vi "configure_scaffold.vi"(8 "error in (no error)":errorcluster, 10 "visibilities":T1, 11 "ScanModeDL090923Scaffold in":refnum<class "ImagingModeDL090923Scaffold.lvclass">) -> (0 "error out":errorcluster, 3 "ScanModeDL090923Scaffold out":refnum<class "ImagingModeDL090923Scaffold.lvclass">)   [LabVIEW 2010, in "ImagingModeDL090923Scaffold.lvclass"]
uses:
  ImagingModeDL090923Scaffold.lvclass
  configuration_visibility_cluster.ctl
  component_configuration_visibility_cluster.ctl
  common/xcontrols/XComponentSpecification/XComponentSpecification/XComponentSpecification.xctl
  ImagingModeDL090923Scaffold.lvclass/ImagingModeDL090923Scaffold.ctl
  Stimulator/GenericStimulator/GenericStimulator/GenericStimulator.lvclass
  Analyser/GenericAnalyser/GenericAnalyser/GenericAnalyser.lvclass
  Display/GenericDisplay/GenericDisplay/GenericDisplay.lvclass
  DataCollection/GenericDataCollection/GenericDataCollection/GenericDataCollection.lvclass
  ImageAssembler/GenericImageAssembler/GenericImageAssembler/GenericImageAssembler.lvclass
  DAQ/GenericDAQ/GenericDAQ/GenericDAQ.lvclass
  ScanHead/GenericScanHead/GenericScanHead/GenericScanHead.lvclass
  Trajectory/GenericTrajectory/GenericTrajectory/GenericTrajectory.lvclass
  Instrument/GenericInstrument/GenericInstrument/GenericInstrument.lvclass
  common/classes/ErrorController/ErrorController/class_data.vi
  common/classes/GenericComponent/GenericComponent/GenericComponent.lvclass
  common/classes/ErrorController/ErrorController/ErrorController.lvclass
panel:
  out "LSID":string
  in  "Tab Control":T3(tab)
  in  "Instrument adapter path":path caption="adapter path"
  in  "instrument spec":T4(xcontrol)
  in  "Trajectory adapter path":path caption="adapter path"
  in  "trajectory spec":T4(xcontrol)
  in  "ScanHead adapter path":path caption="adapter path"
  in  "scanHead spec":T4(xcontrol)
  in  "DAQ adapter path":path caption="adapter path"
  in  "daq spec":T4(xcontrol)
  in  "ImageAssembler adapter path":path caption="adapter path"
  in  "Trajectory-to-ImageAssembler adapter":path caption="trajectory-to-image-assembler adapter (has to be compatible with both the trajectory and the image assembler you have chosen!)"
  in  "imageAssembler spec":T4(xcontrol)
  in  "DataCollection adapter path":path caption="adapter path"
  in  "dataCollection spec":T4(xcontrol)
  in  "Display adapter path":path caption="adapter path"
  in  "display spec":T4(xcontrol)
  in  "Analyser adapter path":path caption="adapter path"
  in  "analyser spec":T4(xcontrol)
  in  "Stimulator adapter path":path caption="adapter path"
  in  "stimulator spec":T4(xcontrol)
  in  "save":bool
  in  "cancel":bool
  out "Configuration":string
  # "Configure ImagingMode"
  # "The ImagingMode component is the central component that determines how images are acquired. It determines also all other top-level components which have to be defined on this configuration dialog (see other tabs)."
  # "The Instrument component can control and/or hold information about accessory devices and hardware component."
  # "In laser-scanning-based imagingModes, the Trajectory component defines how the laser focal point is moved through the sample."
  # "In laser-scanning-based imagingModes, the ScanHead component controls the invididual laser scanners."
  # "The DAQ component is responsible for reading in image data (either as a stream of pixels in laser-scanning-based ImagingModes, or as images in the case of camera-based ImagingModes)."
  # "The ImageAssembler if responsible for assembling pixels streams into whole images and/or refinement of these images."
  # "The DataCollection component is responsible for storing images permanently to disk."
  # "The Display component is responsible for displaying images to the users."
  # "The Analyser component is responsible for analysing image streams. \n\nNote: Leave the input fields below empty if you are not interested in on-line analysis of acquired images."
  # "The Stimulator component can deliver stimuli to the sample being imaged. \n\nNote: leave the input fields below empty if you don't want to control a stimulator device with HelioScan."
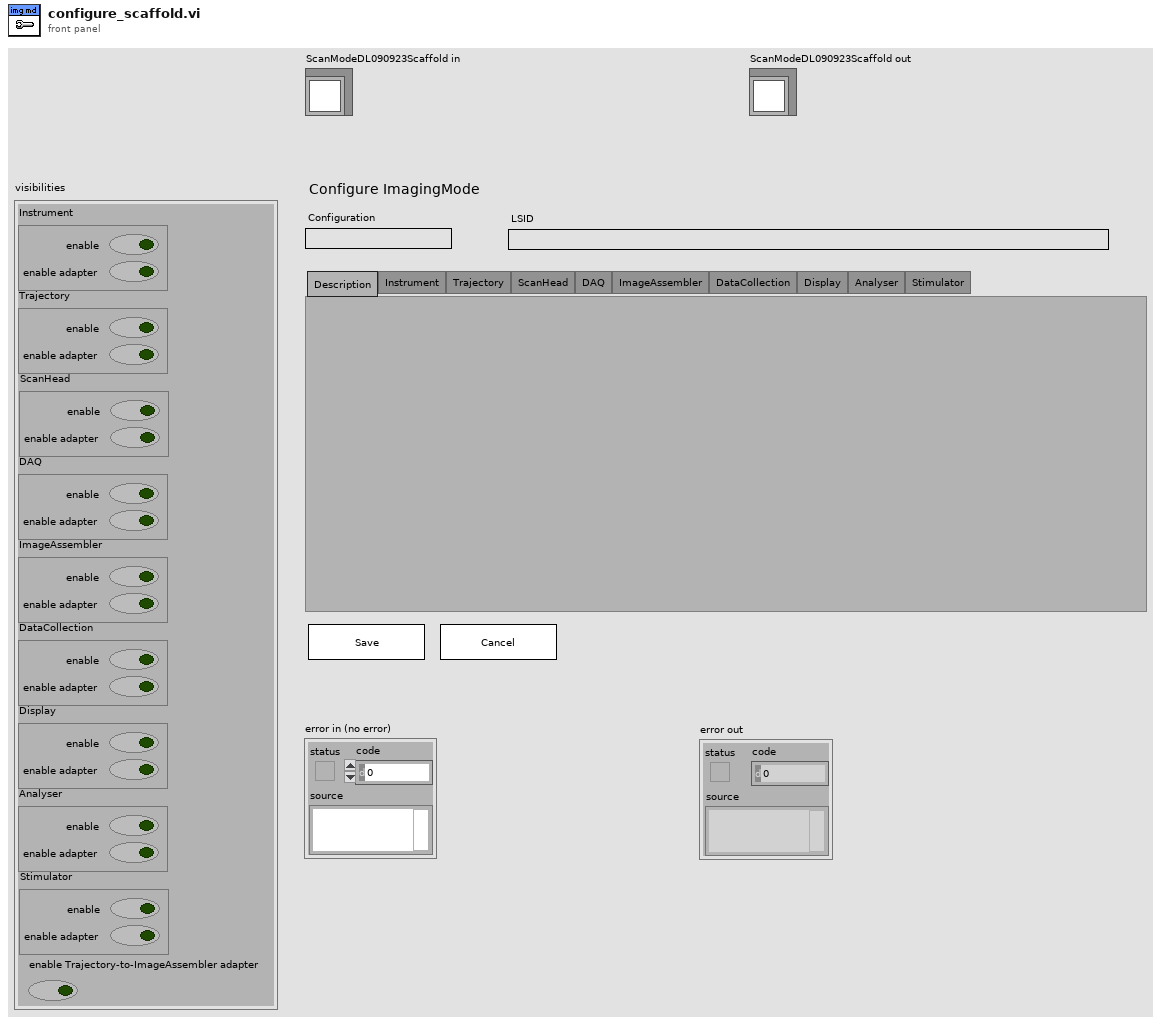
[diagram p1: front panel]
types:
  T1 = typedef "ImagingModeDL090923Scaffold.lvclass/configuration_visibility_cluster.ctl" = cluster{"Instrument":T2, "Trajectory":T2, "ScanHead":T2, "DAQ":T2, "ImageAssembler":T2, "DataCollection":T2, "Display":T2, "Analyser":T2, "Stimulator":T2, "enable Trajectory-to-ImageAssembler adapter":bool}
  T2 = typedef "ImagingModeDL090923Scaffold.lvclass/component_configuration_visibility_cluster.ctl" = cluster{"enable":bool, "enable adapter":bool}
  T3 = enum32{"Description", "Instrument", "Trajectory", "ScanHead", "DAQ", "ImageAssembler", "DataCollection", "Display", "Analyser", "Stimulator"}
  T4 = cluster{"class path":string, "configuration":string, "label":string, "settings name":string}
  T5 = typedef "LSID_cluster.ctl" = cluster{"identifier":string, "revision":i32}
  T6 = typedef "plugin_specification.ctl" = cluster{"class path":string, "configuration":string, "label":string, "settings name":string}
  T7 = typedef "ImagingModeDL090923Scaffold.lvclass/config_data_cluster.ctl" = cluster{"Instrument":T8, "Trajectory":T8, "ScanHead":T8, "DAQ":T8, "ImageAssembler":T8, "DataCollection":T8, "Display":T8, "Analyser":T8, "Stimulator":T8, "Trajectory-to-ImageAssembler adapter path":string, "LSID (cluster)":T5, "special":string}
  T8 = typedef "ImagingModeDL090923Scaffold.lvclass/component_specification_cluster.ctl" = cluster{"specification":T6, "adapter path":string}
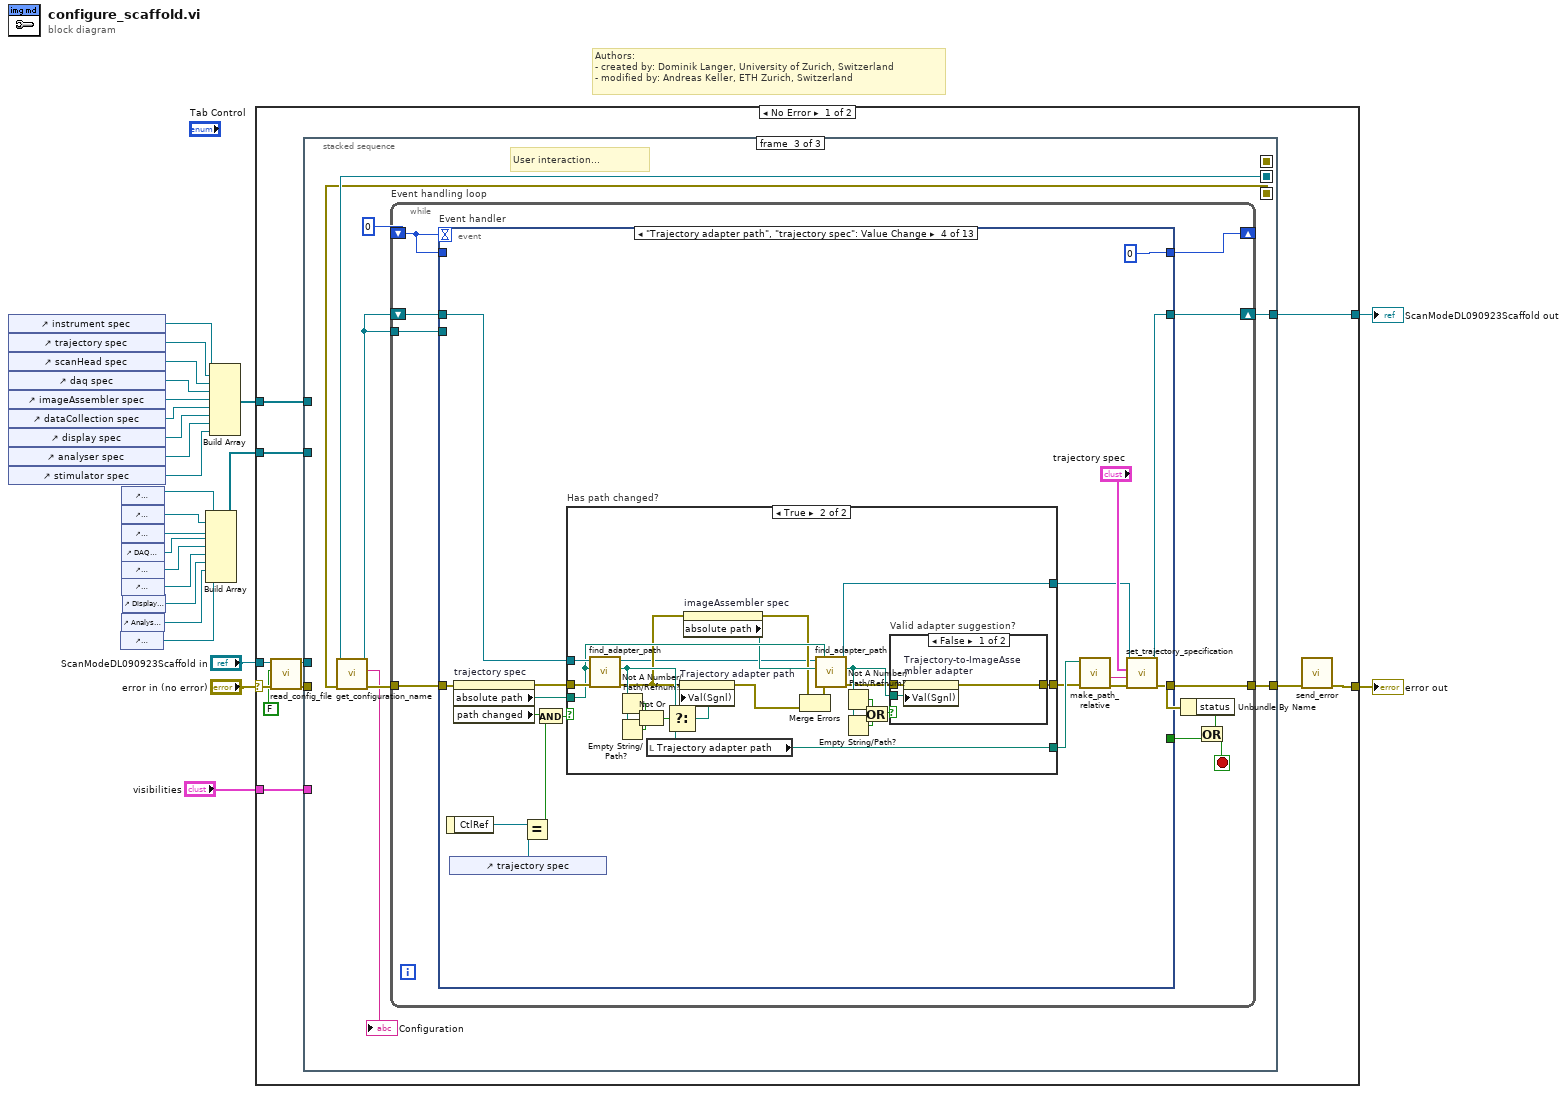
[diagram p0: block diagram]
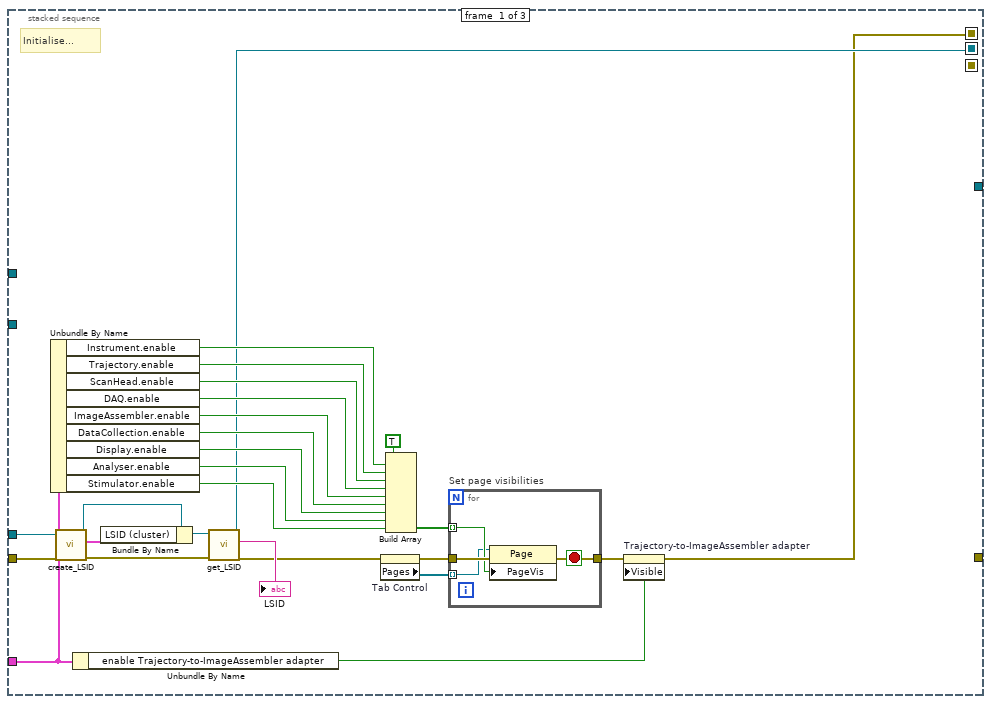
[diagram p2: hidden frame]
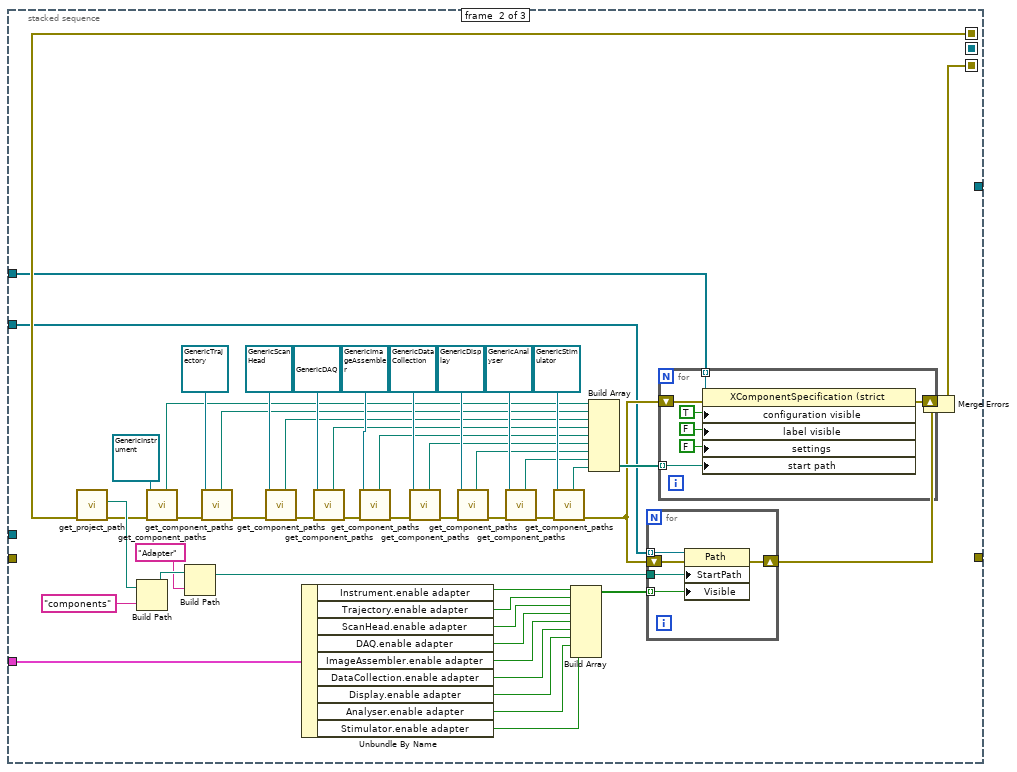
[diagram p3: hidden frame]
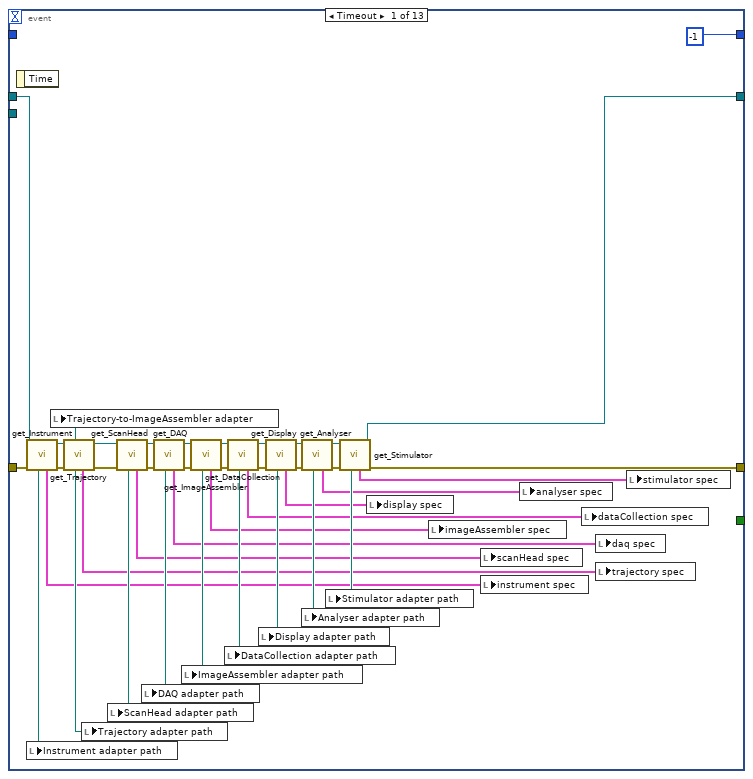
[diagram p4: hidden frame]
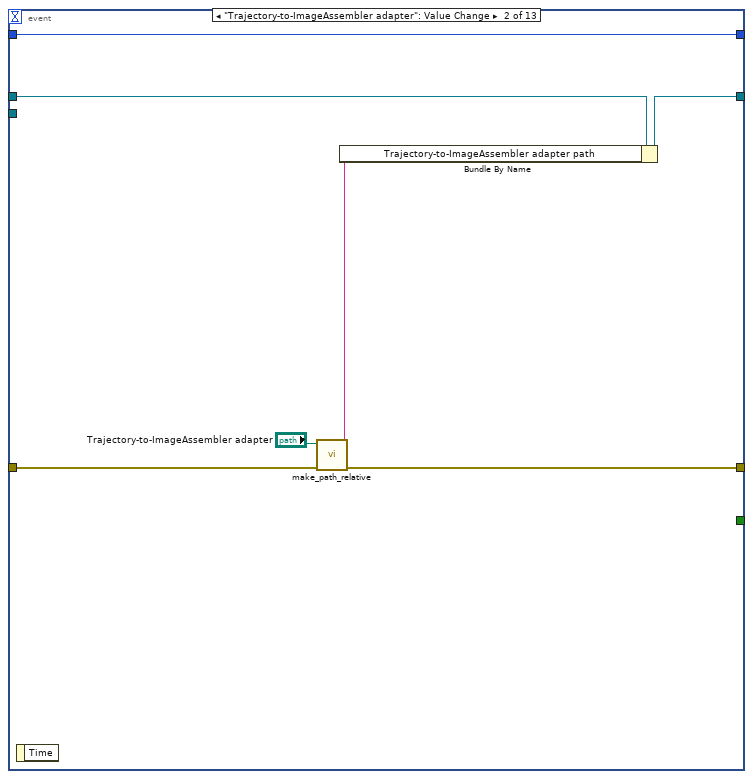
[diagram p5: hidden frame]
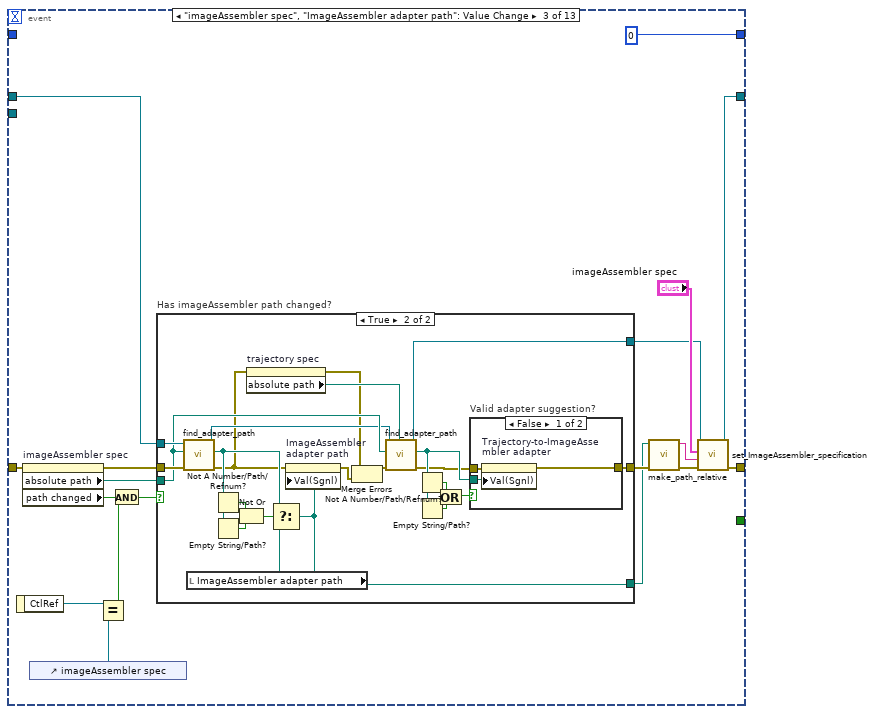
[diagram p6: hidden frame]
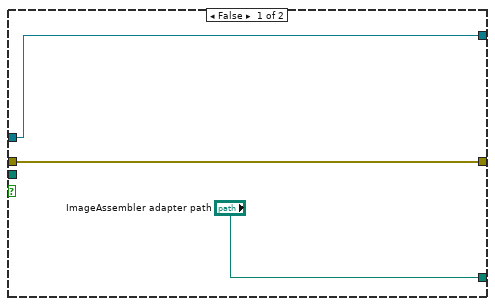
[diagram p7: hidden frame]
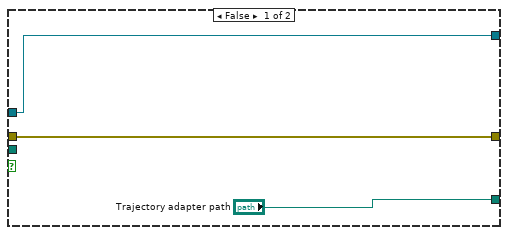
[diagram p9: hidden frame]
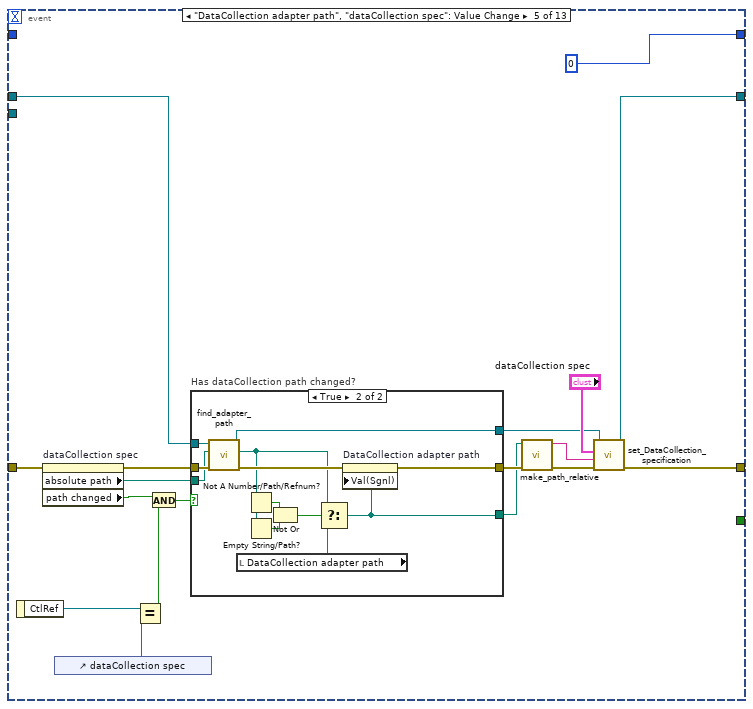
[diagram p11: hidden frame]
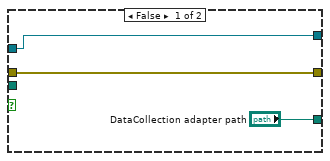
[diagram p12: hidden frame]
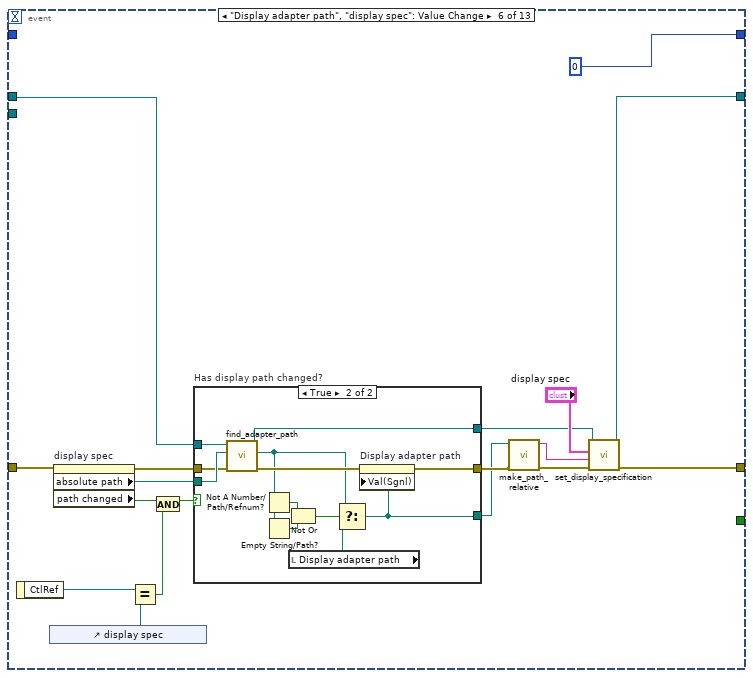
[diagram p13: hidden frame]
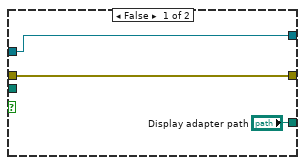
[diagram p14: hidden frame]
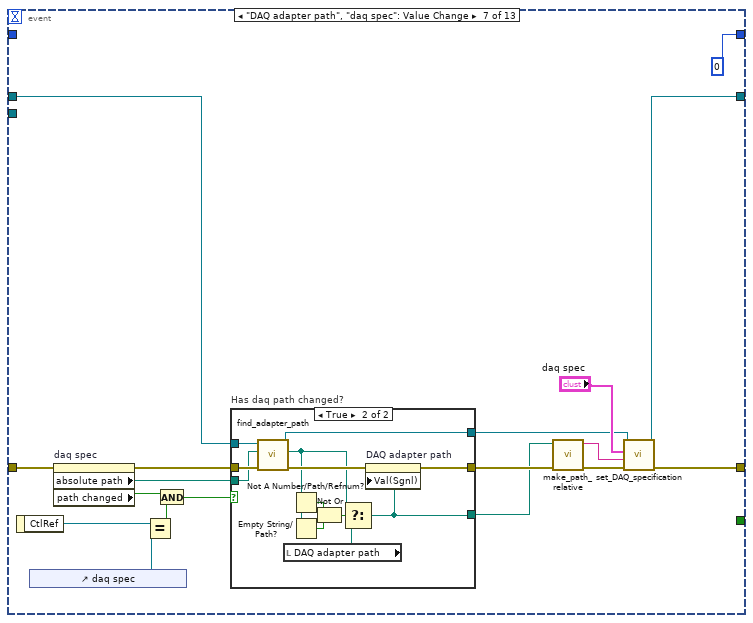
[diagram p15: hidden frame]
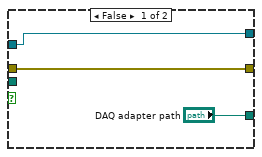
[diagram p16: hidden frame]
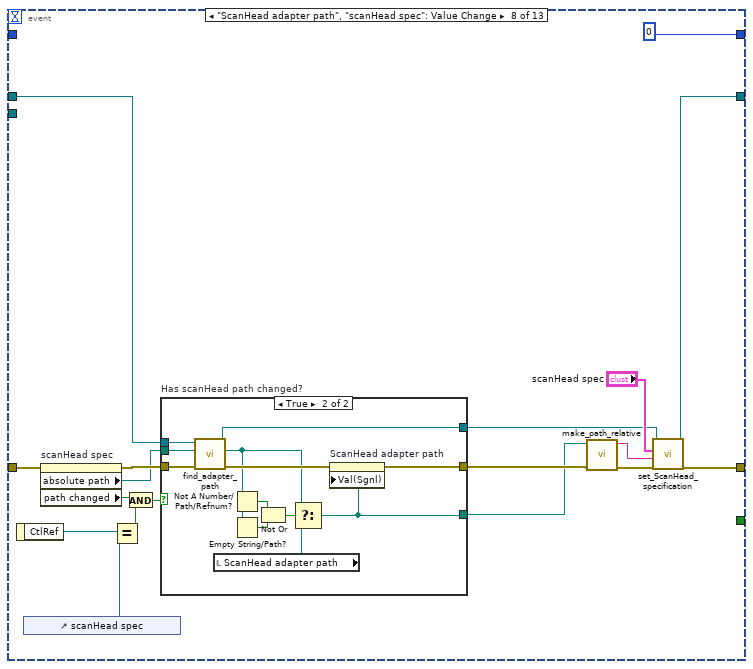
[diagram p17: hidden frame]
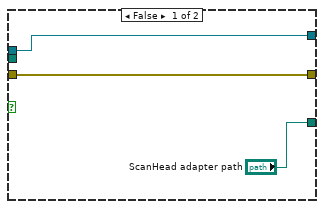
[diagram p18: hidden frame]
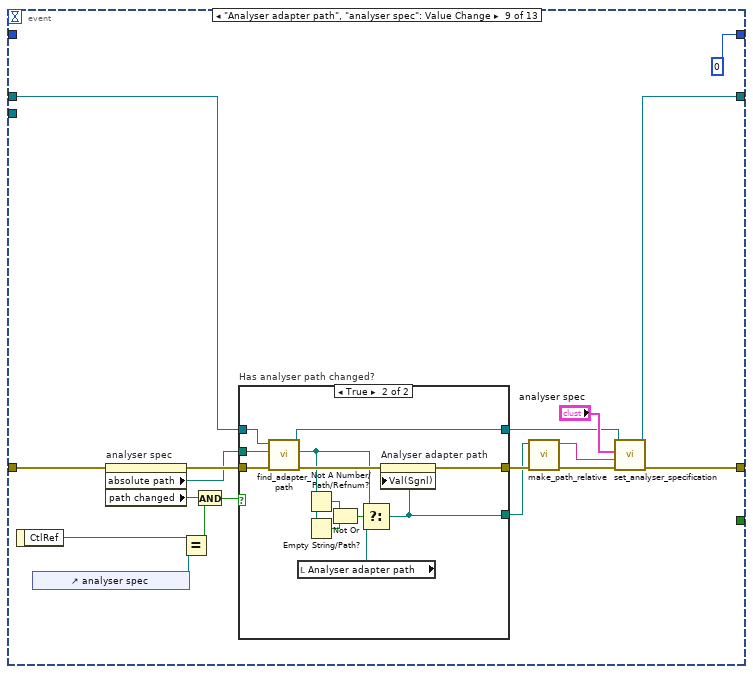
[diagram p19: hidden frame]
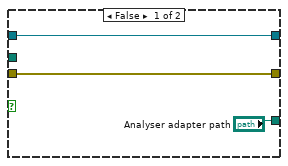
[diagram p20: hidden frame]
diagram:
  # "Authors: \n- created by: Dominik Langer, University of Zurich, Switzerland\n- modified by: Andreas Keller, ETH Zurich, Switzerland"
  n1 = control-ref of="instrument spec"() -> (w18:refnum<vi>)
  n2 = control-ref of="trajectory spec"() -> (w16:refnum<vi>)
  n3 = control-ref of="scanHead spec"() -> (w15:refnum<vi>)
  n4 = control-ref of="daq spec"() -> (w14:refnum<vi>)
  n5 = control-ref of="imageAssembler spec"() -> (w13:refnum<vi>)
  n6 = control-ref of="dataCollection spec"() -> (w12:refnum<vi>)
  n7 = control-ref of="display spec"() -> (w11:refnum<vi>)
  n8 = control-ref of="analyser spec"() -> (w10:refnum<vi>)
  n9 = control-ref of="stimulator spec"() -> (w9:refnum<vi>)
  n10 = control-ref of="Stimulator adapter path"() -> (w2:refnum<vi>)
  n11 = control-ref of="Instrument adapter path"() -> (w20:refnum<vi>)
  n12 = control-ref of="Trajectory adapter path"() -> (w7:refnum<vi>)
  n13 = control-ref of="ScanHead adapter path"() -> (w8:refnum<vi>)
  n14 = control-ref of="DAQ adapter path"() -> (w6:refnum<vi>)
  n15 = control-ref of="ImageAssembler adapter path"() -> (w5:refnum<vi>)
  n16 = control-ref of="DataCollection adapter path"() -> (w4:refnum<vi>)
  n17 = control-ref of="Analyser adapter path"() -> (w1:refnum<vi>)
  n18 = control-ref of="Display adapter path"() -> (w3:refnum<vi>)
  n19 = Build Array(w20, w7, w8, w6, w5, w4, w3, w1, w2) -> (w19:refnum<vi>[])
  n20 = Build Array(w18, w16, w15, w14, w13, w12, w11, w10, w9) -> (w17:refnum<vi>[])
  n21 = case shown="No Error" "error in (no error)" {
    selector: "error in (no error)" -> [w34 w545]
    tunnel: [w29 w545] -> w25
    tunnel: [w36 w544] -> w24
    tunnel: "ScanModeDL090923Scaffold in" -> [w33 w544]
    tunnel: "visibilities" -> [w35 _]
    tunnel: w19 -> [w27 _]
    tunnel: w17 -> [w26 _]
    frame No Error {
      n22 = call-dynamic "read_config_file.vi"("error in (no error)"=w34, "force load?"=FALSE, "GenericPlugin in"=w33) -> ("error out"=w31:errorcluster, "GenericPlugin out"=w32:refnum<class "ImagingModeDL090923Scaffold.lvclass">)  [unwired: 7 in]
      n23 = stacked-sequence {
        seq-local: [w37 _ _] -> [_ w112 _]
        seq-local: [w39 _ _] -> [_ _ w131]
        seq-local: [_ w68 _] -> [_ _ w130]
        tunnel: [_ _ w137] -> w36
        tunnel: w31 -> [w43 _ _]
        tunnel: w32 -> [w41 _ _]
        tunnel: w35 -> [w50 w82 _]
        tunnel: [_ _ w133] -> w28
        tunnel: w27 -> [_ w67 _]
        tunnel: w26 -> [_ w71 _]
        frame #0 {
          # "Initialise..."
          n24 = Unbundle By Name(w50) -> ("Instrument.enable"=w59:bool, "Trajectory.enable"=w58:bool, "ScanHead.enable"=w57:bool, "DAQ.enable"=w56:bool, "ImageAssembler.enable"=w55:bool, "DataCollection.enable"=w54:bool, "Display.enable"=w53:bool, "Analyser.enable"=w52:bool, "Stimulator.enable"=w51:bool)
          n25 = call-dynamic "create_LSID.vi"("error in (no error)"=w43, "GenericPlugin in"=w41) -> ("error out"=w47:errorcluster, "current LSID"=w48:T5, "GenericPlugin out"=w40:refnum<class "ImagingModeDL090923Scaffold.lvclass">)  [unwired: 7 in]
          n26 = Unbundle By Name(w50) -> ("enable Trajectory-to-ImageAssembler adapter"=w49:bool)
          n27 = Bundle By Name(cluster=w40, "LSID (cluster)"=w48) -> (w46:refnum<class "ImagingModeDL090923Scaffold.lvclass">)
          n28 = call-dynamic "get_LSID.vi"("error in (no error)"=w47, "GenericPlugin in"=w46) -> ("error out"=w42:errorcluster, "LSID (string)"=→"LSID":string, "GenericPlugin out"=w39:refnum<class "ImagingModeDL090923Scaffold.lvclass">)  [unwired: 6 in, 1 out]
          n29 = property on="Tab Control" class="TabCtl (strict)"(error in=w42) -> (error out=w62:errorcluster, "Pages"=w61:refnum<vi>[])  [unwired: 1 in, 1 out]
          n30 = Build Array(TRUE ("element"), w59, w58, w57, w56, w55, w54, w53, w52, w51) -> (w60:bool[])
          n31 = for "Set page visibilities" {
            tunnel: w61 -> [w64] mode=indexing
            tunnel: w60 -> [w65] mode=indexing
            tunnel: w62 -> [w66]
            tunnel: [w63] -> w44
            stop <- w63 stop-if-true
            n32 = property class="Page"(reference=w64, error in=w66, "PageVis"=w65) -> (error out=w63:errorcluster)  [unwired: 1 out]
          }
          n33 = property on="Trajectory-to-ImageAssembler adapter" class="Path"(error in=w44, "Visible"=w49) -> (error out=w37:errorcluster)  [unwired: 1 in, 1 out]
        }
        frame #1 {
          n34 = call "get_project_path.vi"("error in (no error)"=w112) -> ("error out"=w111:errorcluster, "helioscan path"=w116:path)  [unwired: 9 in]
          n35 = Build Path(base path=w116, name or relative path="components") -> (appended path=w114:path)
          n36 = call-dynamic "get_component_paths.vi"("error in (no error)"=w111, "GenericComponent in"=refnum<class "GenericInstrument.lvclass"> refnum ("GenericInstrument.lvclass")) -> ("error out"=w109:errorcluster, "component type directory"=w93:path)  [unwired: 4 in, 4 out]
          n37 = Build Path(base path=w114, name or relative path="Adapter") -> (appended path=w94:path)
          n38 = call-dynamic "get_component_paths.vi"("error in (no error)"=w109, "GenericComponent in"=refnum<class "GenericTrajectory.lvclass"> refnum ("GenericTrajectory.lvclass")) -> ("error out"=w107:errorcluster, "component type directory"=w92:path)  [unwired: 4 in, 4 out]
          n39 = call-dynamic "get_component_paths.vi"("error in (no error)"=w107, "GenericComponent in"=refnum<class "GenericScanHead.lvclass"> refnum ("GenericScanHead.lvclass")) -> ("error out"=w106:errorcluster, "component type directory"=w91:path)  [unwired: 4 in, 4 out]
          n40 = Unbundle By Name(w82) -> ("Instrument.enable adapter"=w81:bool, "Trajectory.enable adapter"=w80:bool, "ScanHead.enable adapter"=w79:bool, "DAQ.enable adapter"=w78:bool, "ImageAssembler.enable adapter"=w77:bool, "DataCollection.enable adapter"=w76:bool, "Display.enable adapter"=w75:bool, "Analyser.enable adapter"=w74:bool, "Stimulator.enable adapter"=w73:bool)
          n41 = call-dynamic "get_component_paths.vi"("error in (no error)"=w106, "GenericComponent in"=refnum<class "GenericDAQ.lvclass"> refnum ("GenericDAQ.lvclass")) -> ("error out"=w105:errorcluster, "component type directory"=w90:path)  [unwired: 4 in, 4 out]
          n42 = call-dynamic "get_component_paths.vi"("error in (no error)"=w105, "GenericComponent in"=refnum<class "GenericImageAssembler.lvclass"> refnum ("GenericImageAssembler.lvclass")) -> ("error out"=w104:errorcluster, "component type directory"=w89:path)  [unwired: 4 in, 4 out]
          n43 = call-dynamic "get_component_paths.vi"("error in (no error)"=w104, "GenericComponent in"=refnum<class "GenericDataCollection.lvclass"> refnum ("GenericDataCollection.lvclass")) -> ("error out"=w100:errorcluster, "component type directory"=w88:path)  [unwired: 4 in, 4 out]
          n44 = call-dynamic "get_component_paths.vi"("error in (no error)"=w100, "GenericComponent in"=refnum<class "GenericDisplay.lvclass"> refnum ("GenericDisplay.lvclass")) -> ("error out"=w99:errorcluster, "component type directory"=w87:path)  [unwired: 4 in, 4 out]
          n45 = call-dynamic "get_component_paths.vi"("error in (no error)"=w99, "GenericComponent in"=refnum<class "GenericAnalyser.lvclass"> refnum ("GenericAnalyser.lvclass")) -> ("error out"=w98:errorcluster, "component type directory"=w86:path)  [unwired: 4 in, 4 out]
          n46 = call-dynamic "get_component_paths.vi"("error in (no error)"=w98, "GenericComponent in"=refnum<class "GenericStimulator.lvclass"> refnum ("GenericStimulator.lvclass")) -> ("error out"=w83:errorcluster, "component type directory"=w85:path)  [unwired: 4 in, 4 out]
          n47 = Build Array(w81, w80, w79, w78, w77, w76, w75, w74, w73) -> (w72:bool[])
          n48 = Build Array(w93, w92, w91, w90, w89, w88, w87, w86, w85) -> (w84:path[])
          n49 = for {
            tunnel: w94 -> [w129]
            shift-right: [w126] -> w69
            shift-left: w83 -> [w128]
            tunnel: w67 -> [w127] mode=indexing
            tunnel: w72 -> [w125] mode=indexing
            n50 = property on="Property Node" class="Path"(reference=w127, error in=w128, "StartPath"=w129, "Visible"=w125) -> (error out=w126:errorcluster)  [unwired: 1 out]
          }
          n51 = for {
            tunnel: w84 -> [w121] mode=indexing
            shift-right: [w119] -> w70
            shift-left: w83 -> [w120]
            tunnel: w71 -> [w118] mode=indexing
            n52 = property on="Property Node" class="XComponentSpecification (strict"(reference=w118, error in=w120, "configuration visible"=TRUE, "label visible"=FALSE, "settings"=FALSE ("settings visible"), "start path"=w121) -> (error out=w119:errorcluster)  [unwired: 1 out]
          }
          n53 = Merge Errors(w70, w69) -> (w68:errorcluster)
        }
        frame #2 {
          # "User interaction..."
          n54 = call "get_configuration_name.vi"("error in (no error)"=w130, "GenericPlugin.lvclass in"=w131) -> ("error out"=w135:errorcluster, "configuration name"=→"Configuration":string, "GenericPlugin.lvclass out"=w132:refnum<class "ImagingModeDL090923Scaffold.lvclass">)  [unwired: 7 in]
          n55 = while "Event handling loop" {
            shift-right: [w145] -> w137
            shift-left: w132 -> [w147]
            shift-right: [w144] -> _
            shift-left: 0 -> [w143]
            tunnel: w132 -> [w142]
            tunnel: w135 -> [w146]
            tunnel: [w141] -> w133
            stop <- w138 stop-if-true
            n56 = event "Event handler" shown="[3] \"Trajectory adapter path\", \"trajectory spec\": Value Change" {
              selector: _ -> [_ _ _ _ _ _ _ _ _ _ _ _ _]
              dyn-events: _ -> [_ _ _ _ _ _ _ _ _ _ _ _ _]
              timeout: w143 -> [_ _ _ _ _ _ _ _ _ _ _ _ _]
              tunnel: w147 -> [w160 w192 w203 w248 w296 w330 w361 w394 w430 w461 w493 _ w527]
              tunnel: w146 -> [w175 w191 w206 w253 w298 w333 w364 w399 w428 w464 w498 w523 w529]
              tunnel: [w158 w193 w210 w257 w304 w337 w370 w403 w436 w469 w502 w520 w533] -> w145
              tunnel: [w156 w190 w211 w258 w305 w338 w371 w404 w437 w470 w503 w523 w534] -> w141
              tunnel: [_ _ _ _ _ _ _ _ _ _ _ TRUE TRUE] -> w139
              tunnel: [-1 w194 0 0 0 0 0 0 0 0 0 w521 w532] -> w144
              tunnel: w143 -> [_ w194 _ _ _ _ _ _ _ _ _ w521 w532]
              tunnel: w142 -> [_ _ _ _ _ _ _ _ _ _ _ w520 w525]
              event Timeout {
                n57 = event-data() -> ()  [unwired: 2 out]
                n58 = call-dynamic "get_Instrument.vi"("error in (no error)"=w175, "ScanModeDL090923Scaffold in"=w160) -> ("error out"=w174:errorcluster, "ScanModeDL090923Scaffold out"=w176:refnum<class "ImagingModeDL090923Scaffold.lvclass">, "Instrument specification"=w157:T6, "adapter path"=w181:path)  [unwired: 4 in, 2 out]
                n59 = local write "Instrument adapter path"(w181) -> ()
                n60 = call-dynamic "get_Trajectory.vi"("error in (no error)"=w174, "ScanModeDL090923Scaffold in"=w176) -> ("error out"=w173:errorcluster, "ScanModeDL090923Scaffold out"=w161:refnum<class "ImagingModeDL090923Scaffold.lvclass">, "specification"=w155:T6, "adapter path"=w185:path, "Trajectory-to-ImageAssembler adapter path"=w159:path)  [unwired: 2 in, 3 out]
                n61 = local write "Trajectory-to-ImageAssembler adapter"(w159) -> ()
                n62 = local write "Trajectory adapter path"(w185) -> ()
                n63 = call-dynamic "get_ScanHead.vi"("error in (no error)"=w173, "ScanModeDL090923Scaffold in"=w161) -> ("error out"=w172:errorcluster, "ScanModeDL090923Scaffold out"=w162:refnum<class "ImagingModeDL090923Scaffold.lvclass">, "ScanHead specification"=w154:T6, "adapter path"=w177:path)  [unwired: 4 in, 2 out]
                n64 = local write "ScanHead adapter path"(w177) -> ()
                n65 = call-dynamic "get_DAQ.vi"("error in (no error)"=w172, "ScanModeDL090923Scaffold in"=w162) -> ("error out"=w171:errorcluster, "ScanModeDL090923Scaffold out"=w163:refnum<class "ImagingModeDL090923Scaffold.lvclass">, "DAQ specification"=w153:T6, "adapter path"=w179:path)  [unwired: 4 in, 2 out]
                n66 = local write "DAQ adapter path"(w179) -> ()
                n67 = call-dynamic "get_ImageAssembler.vi"("error in (no error)"=w171, "ScanModeDL090923Scaffold in"=w163) -> ("error out"=w170:errorcluster, "ScanModeDL090923Scaffold out"=w186:refnum<class "ImagingModeDL090923Scaffold.lvclass">, "ImageAssembler specification"=w148:T6, "adapter path"=w184:path)  [unwired: 4 in, 2 out]
                n68 = local write "ImageAssembler adapter path"(w184) -> ()
                n69 = call-dynamic "get_DataCollection.vi"("error in (no error)"=w170, "ScanModeDL090923Scaffold in"=w186) -> ("error out"=w169:errorcluster, "ScanModeDL090923Scaffold out"=w168:refnum<class "ImagingModeDL090923Scaffold.lvclass">, "DataCollection specification"=w149:T6, "adapter path"=w183:path)  [unwired: 4 in, 2 out]
                n70 = local write "DataCollection adapter path"(w183) -> ()
                n71 = call-dynamic "get_Display.vi"("error in (no error)"=w169, "ScanModeDL090923Scaffold in"=w168) -> ("error out"=w166:errorcluster, "ScanModeDL090923Scaffold out"=w167:refnum<class "ImagingModeDL090923Scaffold.lvclass">, "Display specification"=w150:T6, "adapter path"=w178:path)  [unwired: 4 in, 2 out]
                n72 = local write "Display adapter path"(w178) -> ()
                n73 = call-dynamic "get_Analyser.vi"("error in (no error)"=w166, "ScanModeDL090923Scaffold in"=w167) -> ("error out"=w165:errorcluster, "ScanModeDL090923Scaffold out"=w164:refnum<class "ImagingModeDL090923Scaffold.lvclass">, "Analyser specification"=w151:T6, "adapter path"=w180:path)  [unwired: 4 in, 2 out]
                n74 = local write "Analyser adapter path"(w180) -> ()
                n75 = call-dynamic "get_Stimulator.vi"("error in (no error)"=w165, "ScanModeDL090923Scaffold in"=w164) -> ("error out"=w156:errorcluster, "ScanModeDL090923Scaffold out"=w158:refnum<class "ImagingModeDL090923Scaffold.lvclass">, "Stimulator specification"=w152:T6, "adapter path"=w182:path)  [unwired: 4 in, 2 out]
                n76 = local write "Stimulator adapter path"(w182) -> ()
                n77 = local write "display spec"(w150) -> ()
                n78 = local write "imageAssembler spec"(w148) -> ()
                n79 = local write "scanHead spec"(w154) -> ()
                n80 = local write "instrument spec"(w157) -> ()
                n81 = local write "analyser spec"(w151) -> ()
                n82 = local write "dataCollection spec"(w149) -> ()
                n83 = local write "daq spec"(w153) -> ()
                n84 = local write "trajectory spec"(w155) -> ()
                n85 = local write "stimulator spec"(w152) -> ()
              }
              event "Trajectory-to-ImageAssembler adapter": Value Change {
                n86 = event-data() -> ()  [unwired: 2 out]
                n87 = call "make_path_relative.vi"("error in (no error)"=w191, "absolute path"="Trajectory-to-ImageAssembler adapter") -> ("error out"=w190:errorcluster, "relative path"=w189:string)  [unwired: 8 in]
                n88 = Bundle By Name(cluster=w192, "Trajectory-to-ImageAssembler adapter path"=w189) -> (w193:refnum<class "ImagingModeDL090923Scaffold.lvclass">)
              }
              event "imageAssembler spec", "ImageAssembler adapter path": Value Change {
                n89 = event-data() -> ("CtlRef"=w195:refnum<vi>)  [unwired: 1 out]
                n90 = property on="imageAssembler spec" class="XComponentSpecification (strict"(error in=w206) -> (error out=w205:errorcluster, "absolute path"=w204:path, "path changed"=w199:bool)  [unwired: 1 in, 1 out]
                n91 = control-ref of="imageAssembler spec"() -> (w197:refnum<vi>)
                n92 = Equal?(x=w195, y=w197) -> (x = y?=w196:bool)
                n93 = And(x=w199, y=w196) -> (x .and. y?=w198:bool)
                n94 = case "Has imageAssembler path changed?" shown="True" w198 {
                  tunnel: w205 -> [w214 w232]
                  tunnel: w204 -> [_ w223]
                  tunnel: w203 -> [w215 w231]
                  tunnel: [w215 w221] -> w202
                  tunnel: [w214 w224] -> w201
                  tunnel: ["ImageAssembler adapter path" w230] -> w200
                  frame False {
                  }
                  frame True {
                    n95 = call-dynamic "find_adapter_path.vi"("error in (no error)"=w232, "target component path"=w223, "GenericComponent in"=w231) -> ("error out"=w220:errorcluster, "Path"=w234:path, "GenericComponent out"=w222:refnum<class "ImagingModeDL090923Scaffold.lvclass">)  [unwired: 6 in]
                    n96 = local read "ImageAssembler adapter path"() -> (w233:path)
                    n97 = Not A Number/Path/Refnum?(number/path/refnum=w234) -> (NaN/Path/Refnum?=w236:bool)
                    n98 = Empty String/Path?(string/path=w234) -> (empty?=w235:bool)
                    n99 = Not Or(1:w235, 2:w236) -> (0:w237:bool)
                    n100 = property on="trajectory spec" class="XComponentSpecification (strict"(error in=w220) -> (error out=w218:errorcluster, "absolute path"=w219:path)  [unwired: 1 in, 1 out]
                    n101 = Select(t=w234, s=w237, f=w233) -> (s? t:f=w230:path)
                    n102 = property on="ImageAssembler adapter path" class="Path"(error in=w220, "Val(Sgnl)"=w230) -> (error out=w217:errorcluster)  [unwired: 1 in, 1 out]
                    n103 = Merge Errors(w218, w217) -> (w216:errorcluster)
                    n104 = call-dynamic "find_adapter_path.vi"("source component path (if source not provided by object in)"=w219, "error in (no error)"=w216, "target component path"=w223, "GenericComponent in"=w222) -> ("error out"=w228:errorcluster, "Path"=w229:path, "GenericComponent out"=w221:refnum<class "ImagingModeDL090923Scaffold.lvclass">)  [unwired: 5 in]
                    n105 = Not A Number/Path/Refnum?(number/path/refnum=w229) -> (NaN/Path/Refnum?=w225:bool)
                    n106 = Empty String/Path?(string/path=w229) -> (empty?=w226:bool)
                    n107 = Or(x=w225, y=w226) -> (x .or. y?=w227:bool)
                    n108 = case "Valid adapter suggestion?" shown="False" w227 {
                      tunnel: w228 -> [w240 w241]
                      tunnel: [w239 w241] -> w224
                      tunnel: w229 -> [w238 _]
                      frame False {
                        n109 = property on="Trajectory-to-ImageAssembler adapter" class="Path"(error in=w240, "Val(Sgnl)"=w238) -> (error out=w239:errorcluster)  [unwired: 1 in, 1 out]
                      }
                      frame True {
                      }
                    }
                  }
                }
                n110 = call "make_path_relative.vi"("error in (no error)"=w201, "absolute path"=w200) -> ("error out"=w209:errorcluster, "relative path"=w208:string)  [unwired: 8 in]
                n111 = call-dynamic "set_ImageAssembler_specification.vi"("error in (no error)"=w209, "ImageAssembler adapter path"=w208, "ImageAssembler specification"="imageAssembler spec", "ScanModeDL090923Scaffold in"=w202) -> ("error out"=w211:errorcluster, "ScanModeDL090923Scaffold out"=w210:refnum<class "ImagingModeDL090923Scaffold.lvclass">)  [unwired: 6 in]
              }
              event "Trajectory adapter path", "trajectory spec": Value Change {
                n112 = event-data() -> ("CtlRef"=w243:refnum<vi>)  [unwired: 1 out]
                n113 = control-ref of="trajectory spec"() -> (w242:refnum<vi>)
                n114 = property on="trajectory spec" class="XComponentSpecification (strict"(error in=w253) -> (error out=w252:errorcluster, "absolute path"=w249:path, "path changed"=w245:bool)  [unwired: 1 in, 1 out]
                n115 = Equal?(x=w243, y=w242) -> (x = y?=w246:bool)
                n116 = And(x=w245, y=w246) -> (x .and. y?=w244:bool)
                n117 = case "Has path changed?" shown="True" w244 {
                  tunnel: w252 -> [w261 w279]
                  tunnel: ["Trajectory adapter path" w278] -> w251
                  tunnel: [w261 w271] -> w250
                  tunnel: w249 -> [_ w270]
                  tunnel: w248 -> [w260 w277]
                  tunnel: [w260 w263] -> w247
                  frame False {
                  }
                  frame True {
                    n118 = call-dynamic "find_adapter_path.vi"("error in (no error)"=w279, "target component path"=w270, "GenericComponent in"=w277) -> ("error out"=w268:errorcluster, "Path"=w281:path, "GenericComponent out"=w264:refnum<class "ImagingModeDL090923Scaffold.lvclass">)  [unwired: 6 in]
                    n119 = Not A Number/Path/Refnum?(number/path/refnum=w281) -> (NaN/Path/Refnum?=w284:bool)
                    n120 = Empty String/Path?(string/path=w281) -> (empty?=w283:bool)
                    n121 = Not Or(1:w283, 2:w284) -> (0:w282:bool)
                    n122 = local read "Trajectory adapter path"() -> (w278:path)
                    n123 = Select(t=w281, s=w282, f=w278) -> (s? t:f=w280:path)
                    n124 = property on="Trajectory adapter path" class="Path"(error in=w268, "Val(Sgnl)"=w280) -> (error out=w266:errorcluster)  [unwired: 1 in, 1 out]
                    n125 = property on="imageAssembler spec" class="XComponentSpecification (strict"(error in=w268) -> (error out=w267:errorcluster, "absolute path"=w269:path)  [unwired: 1 in, 1 out]
                    n126 = Merge Errors(w267, w266) -> (w265:errorcluster)
                    n127 = call-dynamic "find_adapter_path.vi"("source component path (if source not provided by object in)"=w270, "error in (no error)"=w265, "target component path"=w269, "GenericComponent in"=w264) -> ("error out"=w275:errorcluster, "Path"=w276:path, "GenericComponent out"=w263:refnum<class "ImagingModeDL090923Scaffold.lvclass">)  [unwired: 5 in]
                    n128 = Not A Number/Path/Refnum?(number/path/refnum=w276) -> (NaN/Path/Refnum?=w272:bool)
                    n129 = Empty String/Path?(string/path=w276) -> (empty?=w273:bool)
                    n130 = Or(x=w272, y=w273) -> (x .or. y?=w274:bool)
                    n131 = case "Valid adapter suggestion?" shown="False" w274 {
                      tunnel: w275 -> [w287 w288]
                      tunnel: [w286 w288] -> w271
                      tunnel: w276 -> [w285 _]
                      frame False {
                        n132 = property on="Trajectory-to-ImageAssembler adapter" class="Path"(error in=w287, "Val(Sgnl)"=w285) -> (error out=w286:errorcluster)  [unwired: 1 in, 1 out]
                      }
                      frame True {
                      }
                    }
                  }
                }
                n133 = call "make_path_relative.vi"("error in (no error)"=w250, "absolute path"=w251) -> ("error out"=w256:errorcluster, "relative path"=w255:string)  [unwired: 8 in]
                n134 = call-dynamic "set_trajectory_specification.vi"("error in (no error)"=w256, "Trajectory adapter path"=w255, "Trajectory specification"="trajectory spec", "ScanModeDL090923Scaffold in"=w247) -> ("error out"=w258:errorcluster, "ScanModeDL090923Scaffold out"=w257:refnum<class "ImagingModeDL090923Scaffold.lvclass">)  [unwired: 6 in]
              }
              event "DataCollection adapter path", "dataCollection spec": Value Change {
                n135 = event-data() -> ("CtlRef"=w292:refnum<vi>)  [unwired: 1 out]
                n136 = property on="dataCollection spec" class="XComponentSpecification (strict"(error in=w298) -> (error out=w297:errorcluster, "absolute path"=w294:path, "path changed"=w289:bool)  [unwired: 1 in, 1 out]
                n137 = control-ref of="dataCollection spec"() -> (w291:refnum<vi>)
                n138 = Equal?(x=w292, y=w291) -> (x = y?=w293:bool)
                n139 = And(x=w289, y=w293) -> (x .and. y?=w290:bool)
                n140 = case "Has dataCollection path changed?" shown="True" w290 {
                  tunnel: [w308 w315] -> w301
                  tunnel: ["DataCollection adapter path" w314] -> w300
                  tunnel: w297 -> [w308 w313]
                  tunnel: w296 -> [w307 w312]
                  tunnel: [w307 w311] -> w295
                  tunnel: w294 -> [_ w310]
                  frame False {
                  }
                  frame True {
                    n141 = call-dynamic "find_adapter_path.vi"("error in (no error)"=w313, "target component path"=w310, "GenericComponent in"=w312) -> ("error out"=w321:errorcluster, "Path"=w317:path, "GenericComponent out"=w311:refnum<class "ImagingModeDL090923Scaffold.lvclass">)  [unwired: 6 in]
                    n142 = local read "DataCollection adapter path"() -> (w316:path)
                    n143 = Not A Number/Path/Refnum?(number/path/refnum=w317) -> (NaN/Path/Refnum?=w319:bool)
                    n144 = Empty String/Path?(string/path=w317) -> (empty?=w318:bool)
                    n145 = Not Or(1:w318, 2:w319) -> (0:w320:bool)
                    n146 = Select(t=w317, s=w320, f=w316) -> (s? t:f=w314:path)
                    n147 = property on="DataCollection adapter path" class="Path"(error in=w321, "Val(Sgnl)"=w314) -> (error out=w315:errorcluster)  [unwired: 1 in, 1 out]
                  }
                }
                n148 = call "make_path_relative.vi"("error in (no error)"=w301, "absolute path"=w300) -> ("error out"=w303:errorcluster, "relative path"=w302:string)  [unwired: 8 in]
                n149 = call-dynamic "set_DataCollection_specification.vi"("error in (no error)"=w303, "DataCollection adapter path"=w302, "DataCollection specification"="dataCollection spec", "ScanModeDL090923Scaffold in"=w295) -> ("error out"=w305:errorcluster, "ScanModeDL090923Scaffold out"=w304:refnum<class "ImagingModeDL090923Scaffold.lvclass">)  [unwired: 6 in]
              }
              event "Display adapter path", "display spec": Value Change {
                n150 = event-data() -> ("CtlRef"=w325:refnum<vi>)  [unwired: 1 out]
                n151 = control-ref of="display spec"() -> (w326:refnum<vi>)
                n152 = property on="display spec" class="XComponentSpecification (strict"(error in=w333) -> (error out=w331:errorcluster, "absolute path"=w332:path, "path changed"=w323:bool)  [unwired: 1 in, 1 out]
                n153 = Equal?(x=w325, y=w326) -> (x = y?=w324:bool)
                n154 = And(x=w323, y=w324) -> (x .and. y?=w322:bool)
                n155 = case "Has display path changed?" shown="True" w322 {
                  tunnel: w332 -> [_ w348]
                  tunnel: w331 -> [w341 w347]
                  tunnel: w330 -> [w342 w346]
                  tunnel: [w342 w345] -> w329
                  tunnel: [w341 w344] -> w328
                  tunnel: ["Display adapter path" w343] -> w327
                  frame False {
                  }
                  frame True {
                    n156 = call-dynamic "find_adapter_path.vi"("error in (no error)"=w347, "target component path"=w348, "GenericComponent in"=w346) -> ("error out"=w354:errorcluster, "Path"=w350:path, "GenericComponent out"=w345:refnum<class "ImagingModeDL090923Scaffold.lvclass">)  [unwired: 6 in]
                    n157 = Not A Number/Path/Refnum?(number/path/refnum=w350) -> (NaN/Path/Refnum?=w352:bool)
                    n158 = Empty String/Path?(string/path=w350) -> (empty?=w351:bool)
                    n159 = Not Or(1:w351, 2:w352) -> (0:w353:bool)
                    n160 = local read "Display adapter path"() -> (w349:path)
                    n161 = Select(t=w350, s=w353, f=w349) -> (s? t:f=w343:path)
                    n162 = property on="Display adapter path" class="Path"(error in=w354, "Val(Sgnl)"=w343) -> (error out=w344:errorcluster)  [unwired: 1 in, 1 out]
                  }
                }
                n163 = call "make_path_relative.vi"("error in (no error)"=w328, "absolute path"=w327) -> ("error out"=w336:errorcluster, "relative path"=w335:string)  [unwired: 8 in]
                n164 = call-dynamic "set_display_specification.vi"("error in (no error)"=w336, "Display adapter path"=w335, "Display specification"="display spec", "ScanModeDL090923Scaffold in"=w329) -> ("error out"=w338:errorcluster, "ScanModeDL090923Scaffold out"=w337:refnum<class "ImagingModeDL090923Scaffold.lvclass">)  [unwired: 6 in]
              }
              event "DAQ adapter path", "daq spec": Value Change {
                n165 = event-data() -> ("CtlRef"=w357:refnum<vi>)  [unwired: 1 out]
                n166 = control-ref of="daq spec"() -> (w358:refnum<vi>)
                n167 = property on="daq spec" class="XComponentSpecification (strict"(error in=w364) -> (error out=w363:errorcluster, "absolute path"=w362:path, "path changed"=w355:bool)  [unwired: 1 in, 1 out]
                n168 = Equal?(x=w357, y=w358) -> (x = y?=w359:bool)
                n169 = And(x=w355, y=w359) -> (x .and. y?=w356:bool)
                n170 = case "Has daq path changed?" shown="True" w356 {
                  tunnel: w363 -> [w375 w381]
                  tunnel: [w375 w380] -> w366
                  tunnel: ["DAQ adapter path" w379] -> w365
                  tunnel: w362 -> [_ w378]
                  tunnel: w361 -> [w373 w377]
                  tunnel: [w373 w376] -> w360
                  frame False {
                  }
                  frame True {
                    n171 = call-dynamic "find_adapter_path.vi"("error in (no error)"=w381, "target component path"=w378, "GenericComponent in"=w377) -> ("error out"=w387:errorcluster, "Path"=w385:path, "GenericComponent out"=w376:refnum<class "ImagingModeDL090923Scaffold.lvclass">)  [unwired: 6 in]
                    n172 = local read "DAQ adapter path"() -> (w382:path)
                    n173 = Not A Number/Path/Refnum?(number/path/refnum=w385) -> (NaN/Path/Refnum?=w384:bool)
                    n174 = Empty String/Path?(string/path=w385) -> (empty?=w383:bool)
                    n175 = Not Or(1:w383, 2:w384) -> (0:w386:bool)
                    n176 = Select(t=w385, s=w386, f=w382) -> (s? t:f=w379:path)
                    n177 = property on="DAQ adapter path" class="Path"(error in=w387, "Val(Sgnl)"=w379) -> (error out=w380:errorcluster)  [unwired: 1 in, 1 out]
                  }
                }
                n178 = call "make_path_relative.vi"("error in (no error)"=w366, "absolute path"=w365) -> ("error out"=w369:errorcluster, "relative path"=w368:string)  [unwired: 8 in]
                n179 = call-dynamic "set_DAQ_specification.vi"("error in (no error)"=w369, "DAQ adapter path"=w368, "DAQ specification"="daq spec", "ScanModeDL090923Scaffold in"=w360) -> ("error out"=w371:errorcluster, "ScanModeDL090923Scaffold out"=w370:refnum<class "ImagingModeDL090923Scaffold.lvclass">)  [unwired: 6 in]
              }
              event "ScanHead adapter path", "scanHead spec": Value Change {
                n180 = event-data() -> ("CtlRef"=w389:refnum<vi>)  [unwired: 1 out]
                n181 = control-ref of="scanHead spec"() -> (w388:refnum<vi>)
                n182 = property on="scanHead spec" class="XComponentSpecification (strict"(error in=w399) -> (error out=w398:errorcluster, "absolute path"=w397:path, "path changed"=w391:bool)  [unwired: 1 in, 1 out]
                n183 = Equal?(x=w389, y=w388) -> (x = y?=w392:bool)
                n184 = And(x=w391, y=w392) -> (x .and. y?=w390:bool)
                n185 = case "Has scanHead path changed?" shown="True" w390 {
                  tunnel: w398 -> [w407 w414]
                  tunnel: w397 -> [_ w413]
                  tunnel: [w407 w412] -> w396
                  tunnel: ["ScanHead adapter path" w411] -> w395
                  tunnel: w394 -> [w406 w410]
                  tunnel: [w406 w409] -> w393
                  frame False {
                  }
                  frame True {
                    n186 = call-dynamic "find_adapter_path.vi"("error in (no error)"=w414, "target component path"=w413, "GenericComponent in"=w410) -> ("error out"=w420:errorcluster, "Path"=w416:path, "GenericComponent out"=w409:refnum<class "ImagingModeDL090923Scaffold.lvclass">)  [unwired: 6 in]
                    n187 = local read "ScanHead adapter path"() -> (w415:path)
                    n188 = Not A Number/Path/Refnum?(number/path/refnum=w416) -> (NaN/Path/Refnum?=w418:bool)
                    n189 = Empty String/Path?(string/path=w416) -> (empty?=w417:bool)
                    n190 = Not Or(1:w417, 2:w418) -> (0:w419:bool)
                    n191 = Select(t=w416, s=w419, f=w415) -> (s? t:f=w411:path)
                    n192 = property on="ScanHead adapter path" class="Path"(error in=w420, "Val(Sgnl)"=w411) -> (error out=w412:errorcluster)  [unwired: 1 in, 1 out]
                  }
                }
                n193 = call "make_path_relative.vi"("error in (no error)"=w396, "absolute path"=w395) -> ("error out"=w402:errorcluster, "relative path"=w401:string)  [unwired: 8 in]
                n194 = call-dynamic "set_ScanHead_specification.vi"("error in (no error)"=w402, "ScanHead adapter path"=w401, "ScanHead specification"="scanHead spec", "ScanModeDL090923Scaffold in"=w393) -> ("error out"=w404:errorcluster, "ScanModeDL090923Scaffold out"=w403:refnum<class "ImagingModeDL090923Scaffold.lvclass">)  [unwired: 6 in]
              }
              event "Analyser adapter path", "analyser spec": Value Change {
                n195 = event-data() -> ("CtlRef"=w422:refnum<vi>)  [unwired: 1 out]
                n196 = control-ref of="analyser spec"() -> (w421:refnum<vi>)
                n197 = property on="analyser spec" class="XComponentSpecification (strict"(error in=w428) -> (error out=w427:errorcluster, "absolute path"=w426:path, "path changed"=w424:bool)  [unwired: 1 in, 1 out]
                n198 = Equal?(x=w422, y=w421) -> (x = y?=w425:bool)
                n199 = And(x=w424, y=w425) -> (x .and. y?=w423:bool)
                n200 = case "Has analyser path changed?" shown="True" w423 {
                  tunnel: [w439 w447] -> w432
                  tunnel: ["Analyser adapter path" w446] -> w431
                  tunnel: w430 -> [w441 w445]
                  tunnel: [w441 w444] -> w429
                  tunnel: w427 -> [w439 w443]
                  tunnel: w426 -> [_ w442]
                  frame False {
                  }
                  frame True {
                    n201 = call-dynamic "find_adapter_path.vi"("error in (no error)"=w443, "target component path"=w442, "GenericComponent in"=w445) -> ("error out"=w453:errorcluster, "Path"=w449:path, "GenericComponent out"=w444:refnum<class "ImagingModeDL090923Scaffold.lvclass">)  [unwired: 6 in]
                    n202 = local read "Analyser adapter path"() -> (w448:path)
                    n203 = Not A Number/Path/Refnum?(number/path/refnum=w449) -> (NaN/Path/Refnum?=w451:bool)
                    n204 = Empty String/Path?(string/path=w449) -> (empty?=w450:bool)
                    n205 = Not Or(1:w450, 2:w451) -> (0:w452:bool)
                    n206 = Select(t=w449, s=w452, f=w448) -> (s? t:f=w446:path)
                    n207 = property on="Analyser adapter path" class="Path"(error in=w453, "Val(Sgnl)"=w446) -> (error out=w447:errorcluster)  [unwired: 1 in, 1 out]
                  }
                }
                n208 = call "make_path_relative.vi"("error in (no error)"=w432, "absolute path"=w431) -> ("error out"=w435:errorcluster, "relative path"=w434:string)  [unwired: 8 in]
                n209 = call-dynamic "set_analyser_specification.vi"("error in (no error)"=w435, "Analyser adapter path"=w434, "Analyser specification"="analyser spec", "ScanModeDL090923Scaffold in"=w429) -> ("error out"=w437:errorcluster, "ScanModeDL090923Scaffold out"=w436:refnum<class "ImagingModeDL090923Scaffold.lvclass">)  [unwired: 6 in]
              }
              event "Instrument adapter path", "instrument spec": Value Change {
                n210 = event-data() -> ("CtlRef"=w455:refnum<vi>)  [unwired: 1 out]
                n211 = control-ref of="instrument spec"() -> (w454:refnum<vi>)
                n212 = property on="instrument spec" class="XComponentSpecification (strict"(error in=w464) -> (error out=w463:errorcluster, "absolute path"=w462:path, "path changed"=w457:bool)  [unwired: 1 in, 1 out]
                n213 = Equal?(x=w455, y=w454) -> (x = y?=w458:bool)
                n214 = And(x=w457, y=w458) -> (x .and. y?=w456:bool)
                n215 = case "Path changed?" shown="True" w456 {
                  tunnel: [w474 w480] -> w466
                  tunnel: w463 -> [w474 w479]
                  tunnel: w462 -> [_ w478]
                  tunnel: w461 -> [w472 w477]
                  tunnel: [w472 w476] -> w460
                  tunnel: ["Instrument adapter path" w475] -> w459
                  frame False {
                  }
                  frame True {
                    n216 = call-dynamic "find_adapter_path.vi"("error in (no error)"=w479, "target component path"=w478, "GenericComponent in"=w477) -> ("error out"=w486:errorcluster, "Path"=w484:path, "GenericComponent out"=w476:refnum<class "ImagingModeDL090923Scaffold.lvclass">)  [unwired: 6 in]
                    n217 = Not A Number/Path/Refnum?(number/path/refnum=w484) -> (NaN/Path/Refnum?=w482:bool)
                    n218 = Empty String/Path?(string/path=w484) -> (empty?=w483:bool)
                    n219 = Not Or(1:w483, 2:w482) -> (0:w485:bool)
                    n220 = local read "Instrument adapter path"() -> (w481:path)
                    n221 = Select(t=w484, s=w485, f=w481) -> (s? t:f=w475:path)
                    n222 = property on="Instrument adapter path" class="Path"(error in=w486, "Val(Sgnl)"=w475) -> (error out=w480:errorcluster)  [unwired: 1 in, 1 out]
                  }
                }
                n223 = call "make_path_relative.vi"("error in (no error)"=w466, "absolute path"=w459) -> ("error out"=w468:errorcluster, "relative path"=w467:string)  [unwired: 8 in]
                n224 = call-dynamic "set_Instrument_specification.vi"("error in (no error)"=w468, "Instrument adapter path"=w467, "Instrument specification"="instrument spec", "ScanModeDL090923Scaffold in"=w460) -> ("error out"=w470:errorcluster, "ScanModeDL090923Scaffold out"=w469:refnum<class "ImagingModeDL090923Scaffold.lvclass">)  [unwired: 6 in]
              }
              event "Stimulator adapter path", "stimulator spec": Value Change {
                n225 = event-data() -> ("CtlRef"=w488:refnum<vi>)  [unwired: 1 out]
                n226 = control-ref of="stimulator spec"() -> (w487:refnum<vi>)
                n227 = property on="stimulator spec" class="XComponentSpecification (strict"(error in=w498) -> (error out=w497:errorcluster, "absolute path"=w496:path, "path changed"=w490:bool)  [unwired: 1 in, 1 out]
                n228 = Equal?(x=w488, y=w487) -> (x = y?=w491:bool)
                n229 = And(x=w490, y=w491) -> (x .and. y?=w489:bool)
                n230 = case "Has stimulator path changed?" shown="True" w489 {
                  tunnel: w497 -> [w507 w513]
                  tunnel: w496 -> [_ w512]
                  tunnel: [w507 w511] -> w495
                  tunnel: ["Stimulator adapter path" w510] -> w494
                  tunnel: w493 -> [w505 w509]
                  tunnel: [w505 w508] -> w492
                  frame False {
                  }
                  frame True {
                    n231 = call-dynamic "find_adapter_path.vi"("error in (no error)"=w513, "target component path"=w512, "GenericComponent in"=w509) -> ("error out"=w519:errorcluster, "Path"=w515:path, "GenericComponent out"=w508:refnum<class "ImagingModeDL090923Scaffold.lvclass">)  [unwired: 6 in]
                    n232 = Not A Number/Path/Refnum?(number/path/refnum=w515) -> (NaN/Path/Refnum?=w517:bool)
                    n233 = Empty String/Path?(string/path=w515) -> (empty?=w516:bool)
                    n234 = local read "Stimulator adapter path"() -> (w514:path)
                    n235 = Not Or(1:w516, 2:w517) -> (0:w518:bool)
                    n236 = Select(t=w515, s=w518, f=w514) -> (s? t:f=w510:path)
                    n237 = property on="Stimulator adapter path" class="Path"(error in=w519, "Val(Sgnl)"=w510) -> (error out=w511:errorcluster)  [unwired: 1 in, 1 out]
                  }
                }
                n238 = call "make_path_relative.vi"("error in (no error)"=w495, "absolute path"=w494) -> ("error out"=w501:errorcluster, "relative path"=w500:string)  [unwired: 8 in]
                n239 = call-dynamic "set_stimulator_specification.vi"("error in (no error)"=w501, "Stimulator adapter path"=w500, "Stimulator specification"="stimulator spec", "ScanModeDL090923Scaffold in"=w492) -> ("error out"=w503:errorcluster, "ScanModeDL090923Scaffold out"=w502:refnum<class "ImagingModeDL090923Scaffold.lvclass">)  [unwired: 6 in]
              }
              event "cancel": Value Change; Panel Close {
                n240 = event-data() -> ()  [unwired: 2 out]
              }
              event "save": Value Change {
                n241 = event-data() -> ()  [unwired: 2 out]
                n242 = Unbundle By Name(w527) -> ("config data"=w531:T7)
                n243 = Unbundle By Name(w525) -> ("config data"=w526:T7)
                n244 = Not Equal?(x=w526, y=w531) -> (x != y?=w530:bool)
                n245 = case "Anything changed?" shown="False" w530 {
                  tunnel: w529 -> [w537 w543]
                  tunnel: [w537 w542] -> w528
                  tunnel: w527 -> [_ w541]
                  tunnel: [w536 w539] -> w524
                  tunnel: w525 -> [w536 _]
                  frame False {
                  }
                  frame True {
                    n246 = call-dynamic "increase_revision.vi"("error in (no error)"=w543, "GenericPlugin in"=w541) -> ("error out"=w542:errorcluster, "new LSID"=w538:T5, "GenericPlugin out"=w540:refnum<class "ImagingModeDL090923Scaffold.lvclass">)  [unwired: 7 in]
                    n247 = Bundle By Name(cluster=w540, "LSID (cluster)"=w538) -> (w539:refnum<class "ImagingModeDL090923Scaffold.lvclass">)
                  }
                }
                n248 = call-dynamic "save_config_file.vi"("error in (no error)"=w528, "GenericPlugin in"=w524) -> ("error out"=w534:errorcluster, "GenericPlugin out"=w533:refnum<class "ImagingModeDL090923Scaffold.lvclass">)  [unwired: 2 in, 6 out]
              }
            }
            n249 = Unbundle By Name(w141) -> ("status"=w140:bool)
            n250 = Or(x=w140, y=w139) -> (x .or. y?=w138:bool)
          }
        }
      }
      n251 = call "send_error.vi"("error in (no error)"=w28) -> ("error out"=w29:errorcluster)  [unwired: 10 in]
    }
    frame Error {
    }
  }
  "error out" <- w25
  "ScanModeDL090923Scaffold out" <- w24
